vi "PH_Beckhoff_PPMA-Rods.declare digital InputTags.vi"(0 "Instance Name":string="<Instance Name>") -> (1 "Description":string, 2 "Digital Inputs":T2)   [LabVIEW 2014, in "PH_Beckhoff_PPMA-Rods.lvlib"]
uses:
  PH_Beckhoff_PPMA-Rods.lvlib
  PH_Beckhoff/PH_Beckhoff.Digital Inputs.ctl
  PH_Beckhoff_PPMA-Rods.Rods Tags.ctl
  PH_Beckhoff/PH_Beckhoff.lvlib
panel:
  in  "Digital Input Value":T1
  out "Right Size?":bool
  # "Let this VI run to check the size!"
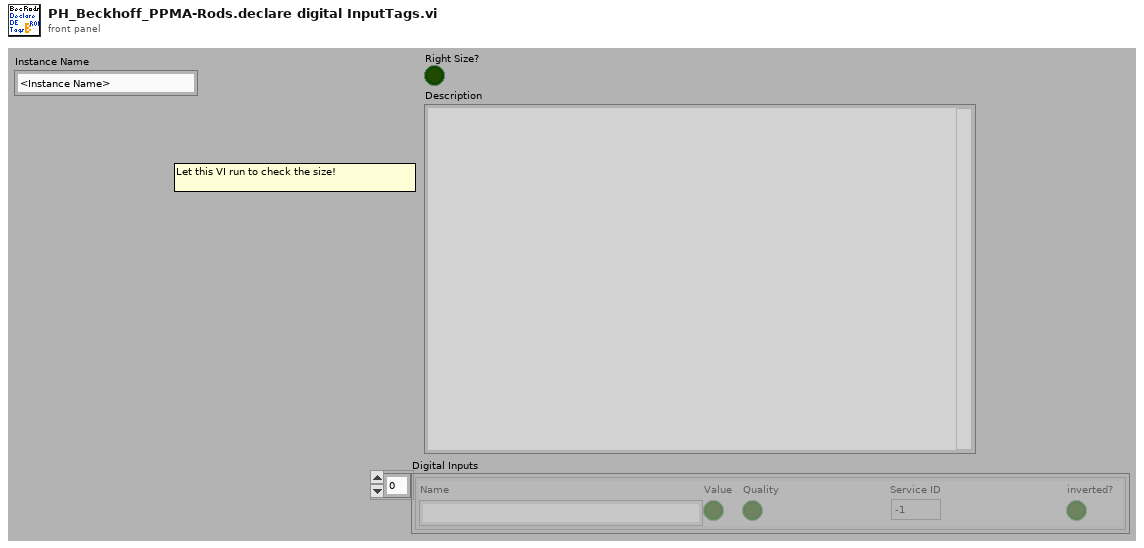
[diagram p1: front panel]
types:
  T1 = cluster{"Name":string, "Value":bool, "Quality":bool, "Service ID":i32, "inverted?":bool}
  T2 = typedef "PH_Beckhoff.lvlib/PH_Beckhoff.Digital Inputs.ctl" = cluster{"Name":string, "Value":bool, "Quality":bool, "Service ID":i32, "inverted?":bool}[]
  T3 = typedef "PH_Beckhoff_PPMA-Rods.lvlib/PH_Beckhoff_PPMA-Rods.Rods Tags.ctl" = enum16{"Rod-up", "earth-ok", "door-locked-K1", "door-locked-K2", "watervalve-closed", "Rods-Chain-A-up", "Rods-Chain-B-up", "HV-Warnlamp-orange", "HV-Warnlamp-green", "Status-Rods-PU-1", "Status-Rods-PU-2", "Status-Rods-PU-3", "Status-Rods-PU-4", "Status-Rods-PU-5", "Status-Rods-PU-6", "Status-Rods-PU-7", "Status-Rods-PU-8", "Status-Rods-PU-9", "Status-Rods-PU-10", "Status-Rods-FR", "Status-Rods-PILC"}
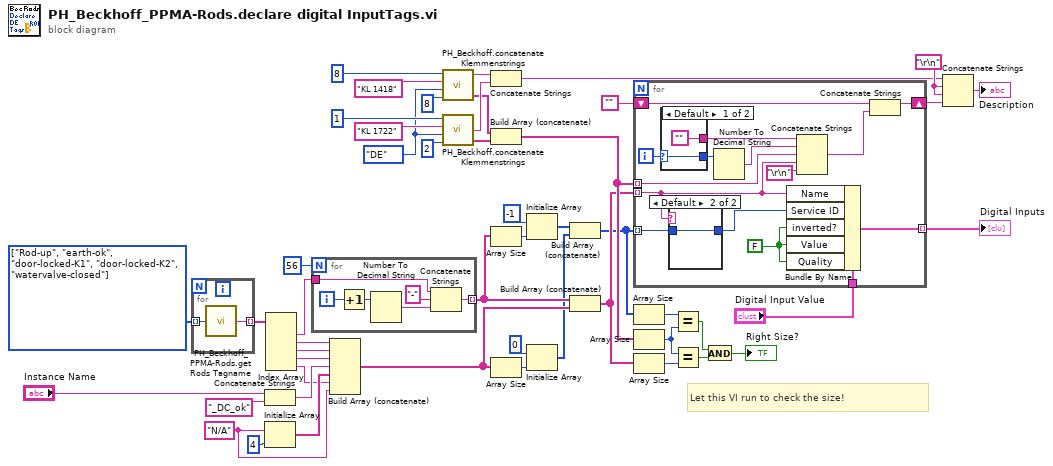
[diagram p0: block diagram]
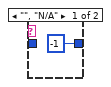
[diagram p2: hidden frame]
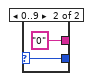
[diagram p3: hidden frame]
diagram:
  w17 = "N/A"
  w29 = T3[] [enum."Rod-up", enum."earth-ok", enum."door-locked-K1", enum."door-locked-K2", enum."watervalve-closed"] items=["Rod-up", "earth-ok", "door-locked-K1", "door-locked-K2", "watervalve-closed", "Rods-Chain-A-up", "Rods-Chain-B-up", "HV-Warnlamp-orange", "HV-Warnlamp-green", "Status-Rods-PU-1", "Status-Rods-PU-2", "Status-Rods-PU-3", "Status-Rods-PU-4", "Status-Rods-PU-5", "Status-Rods-PU-6", "Status-Rods-PU-7", "Status-Rods-PU-8", "Status-Rods-PU-9", "Status-Rods-PU-10", "Status-Rods-FR", "Status-Rods-PILC"]
  w30 = enum16{"AE", "AA", "DE", "DA", "SE"}."DE" ("Type")
  w49 = "\r\n"
  # "Let this VI run to check the size!"
  n1 = for {
    tunnel: w29 -> [w51] mode=indexing
    tunnel: [w50] -> w28 mode=indexing
    n2 = call "PH_Beckhoff_PPMA-Rods.get Rods Tagname.vi"("Rods Tag"=w51) -> ("Rods Tagname"=w50:string)
  }
  n3 = Concatenate Strings("Instance Name", "_DC_ok" ("string")) -> (w21:string)
  n4 = Initialize Array(w17, 4 ("dimension size")) -> (w19:string[])
  n5 = Index Array(array=w28) -> (element #1=w27:string, element #2=w26:string, element #3=w25:string, element #4=w24:string, element #5=w18:string)  [unwired: 5 in]
  n6 = for {
    N: 56 -> [_]
    tunnel: w27 -> [w54]
    tunnel: [w52] -> w9 mode=indexing
    i -> [w57]
    n7 = Increment(x=w57) -> (x+1=w56:i32)
    n8 = Number To Decimal String(number=w56) -> (decimal integer string=w55:string)  [unwired: 1 in]
    n9 = Concatenate Strings(w54, "-" ("string"), w55) -> (w52:string)
  }
  n10 = Build Array (concatenate)(w26, w25, w24, w21, w19, w18, w17) -> (w14:string[])
  n11 = call "PH_Beckhoff.concatenate Klemmenstrings.vi"("# of In- or Outputs"=8, "Type"=w30, "Klemmenname"="KL 1418", "Quantity"=8) -> ("concatenated string array"=w35:string[], "\"<Type>: <Quantity> x <Klemmenname>\""=w37:string)  [unwired: 1 out]
  n12 = call "PH_Beckhoff.concatenate Klemmenstrings.vi"("# of In- or Outputs"=2, "Type"=w30, "Klemmenname"="KL 1722", "Quantity"=1 ("size(s)")) -> ("concatenated string array"=w34:string[], "\"and <Quantity> x <Klemmenname>\""=w36:string)  [unwired: 1 out]
  n13 = Concatenate Strings(w37, w36) -> (w31:string)
  n14 = Build Array (concatenate)(w35, w34) -> (w46:string[])
  n15 = Array Size(array=w9) -> (size(s)=w11:i32)
  n16 = Array Size(array=w14) -> (size(s)=w13:i32)
  n17 = Initialize Array(-1, w11) -> (w8:i32[])
  n18 = Initialize Array(0, w13) -> (w7:i32[])
  n19 = Build Array (concatenate)(w8, w7) -> (w6:i32[])
  n20 = Build Array (concatenate)(w9, w14) -> (w15:string[])
  n21 = for {
    tunnel: w15 -> [w62] mode=indexing
    tunnel: w46 -> [w68] mode=indexing
    shift-right: [w66] -> w47
    shift-left: "" -> [w65]
    tunnel: "Digital Input Value" -> [w64]
    tunnel: [w61] -> w42 mode=indexing
    tunnel: w6 -> [w58] mode=indexing
    i -> [w72]
    w60 = FALSE ("Quality")
    n22 = case shown="Default" w72 {
      selector: w72 -> [w75 w78]
      tunnel: [w75 w78] -> w71
      tunnel: ["" "0"] -> w70
      frame Default {
      }
      frame 0..9 {
      }
    }
    n23 = case shown="Default" w62 {
      tunnel: [-1 w74] -> w63
      tunnel: w58 -> [_ w74]
      frame "", "N/A" {
      }
      frame Default {
      }
    }
    n24 = Number To Decimal String(number=w71) -> (decimal integer string=w69:string)  [unwired: 1 in]
    n25 = Bundle By Name(cluster=w64, "Name"=w62, "Service ID"=w63, "inverted?"=w60, "Value"=w60, "Quality"=w60) -> (w61:T1)
    n26 = Concatenate Strings(w70, w69, w68, w62, "\r\n") -> (w67:string)
    n27 = Concatenate Strings(w65, w67) -> (w66:string)
  }
  "Digital Inputs" <- w42
  n28 = Array Size(array=w6) -> (size(s)=w5:i32)
  n29 = Array Size(array=w46) -> (size(s)=w4:i32)
  n30 = Array Size(array=w15) -> (size(s)=w44:i32)
  n31 = Equal?(x=w5, y=w4) -> (x = y?=w1:bool)
  n32 = Equal?(x=w4, y=w44) -> (x = y?=w2:bool)
  n33 = And(x=w1, y=w2) -> (x .and. y?=→"Right Size?":bool)
  n34 = Concatenate Strings(w31, w49, w49, w47) -> (→"Description":string)
